vi "Fixed Bug.vi"(11 "cluster in":T1) -> (3 "cluster out":T1)   [LabVIEW 2026]
uses:
  Type Defs/Handler Data.ctl
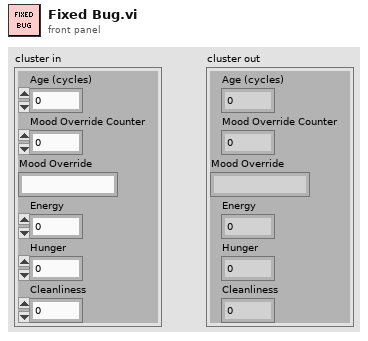
[diagram p1: front panel]
types:
  T1 = typedef "Handler Data.ctl" = cluster{"Age (cycles)":u32, "Mood Override Counter":u32, "Mood Override":string, "Energy":i16, "Hunger":i16, "Cleanliness":i16}
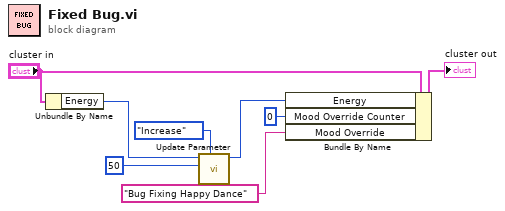
[diagram p0: block diagram]
diagram:
  n1 = Unbundle By Name("cluster in") -> ("Energy"=w3:i16)
  n2 = call "Update Parameter.vi"("Action"=enum16{"Increase", "Decrease"}."Increase", "Modifier"=i16 50 ("y"), "Parameter"=w3) -> ("New Value"=w5:i16)  [unwired: 8 in]
  n3 = Bundle By Name(cluster="cluster in", "Energy"=w5, "Mood Override Counter"=u32 0, "Mood Override"="Bug Fixing Happy Dance") -> (→"cluster out":T1)
